vi "AutoCamCalibration.vi"   [LabVIEW 2019]
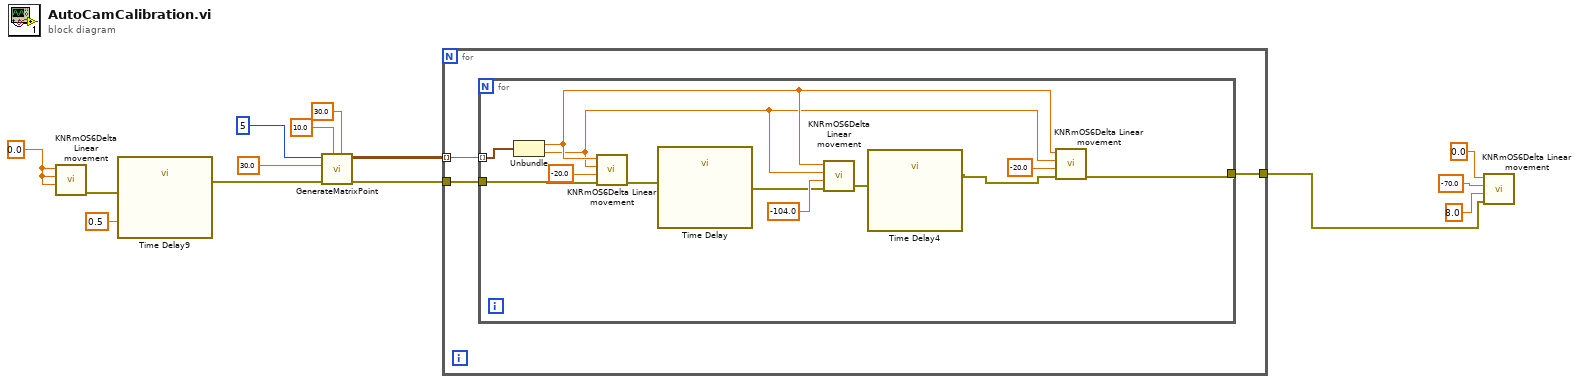
[diagram p0: block diagram]
diagram:
  w11 = 0.0 ("x0")
  n1 = call "KNRmOS6Delta Linear movement.vi"("z0"=w11, "y0"=w11, "x0"=w11) -> ("error out"=w10:errorcluster)  [unwired: 8 in]
  n2 = call "Time Delay9"("error in (no error)"=w10, "Delay Time (s)"=0.5) -> ("error out"=w9:errorcluster)  [unwired: 9 in]
  n3 = call "GenerateMatrixPoint.vi"("YOffSet"=30.0, "XOffSet"=10.0, "error in (no error)"=w9, "Pitch"=30.0, "MatrixSize"=5) -> ("error out"=w4:errorcluster, "MatrixPoint"=w3:cluster{dbl, dbl}[][])  [unwired: 5 in]
  n4 = for {
    tunnel: w4 -> [w17]
    tunnel: w3 -> [w15] mode=indexing
    tunnel: [w16] -> w2
    n5 = for {
      tunnel: w17 -> [w27]
      tunnel: [w20] -> w16
      tunnel: w15 -> [w25] mode=indexing
      n6 = Unbundle(w25) -> (w19:dbl, w18:dbl)
      n7 = call "KNRmOS6Delta Linear movement.vi"("error in (no error)"=w27, "z0"=-20.0, "y0"=w18, "x0"=w19) -> ("error out"=w24:errorcluster)  [unwired: 7 in]
      n8 = call "Time Delay"("error in (no error)"=w24) -> ("error out"=w23:errorcluster)  [unwired: 10 in]
      n9 = call "KNRmOS6Delta Linear movement.vi"("error in (no error)"=w23, "z0"=-104.0, "y0"=w18, "x0"=w19) -> ("error out"=w26:errorcluster)  [unwired: 7 in]
      n10 = call "Time Delay4"("error in (no error)"=w26) -> ("error out"=w21:errorcluster)  [unwired: 10 in]
      n11 = call "KNRmOS6Delta Linear movement.vi"("error in (no error)"=w21, "z0"=-20.0, "y0"=w18, "x0"=w19) -> ("error out"=w20:errorcluster)  [unwired: 7 in]
    }
  }
  n12 = call "KNRmOS6Delta Linear movement.vi"("error in (no error)"=w2, "z0"=8.0, "y0"=-70.0, "x0"=0.0) -> ()  [unwired: 7 in, 1 out]
